vi "Filters_on_Single_Frame_Displacements-2.vi"(5 "[IN] Possibly\nMoving (X,Y)":dbl[][](array[numeric]), 6 "Areas of\nobjects":dbl[][](array[numeric]), 7 "[IN] Primary \nCoordinates (X,Y)":dbl[][](array[numeric]), 8 "error IN":errorcluster, 9 "% DIfference between \nParticle Squares":dbl, 10 "[IN] Dot matrix with \nstatuses for  potentially \nmoving dots":i16[][](array[numeric]), 11 "[IN] Potential\ndisplacement \n(X,Y,dX,dY)":dbl[][](array[numeric])) -> (0 "error OUT":errorcluster, 2 "[OUT] Dot matrix with \nstatuses for potentially \nmoving dots":i16[][](array[numeric]), 3 "[OUT] Filtered\ndisplacements":dbl[][](array[numeric]))   [LabVIEW 2013]
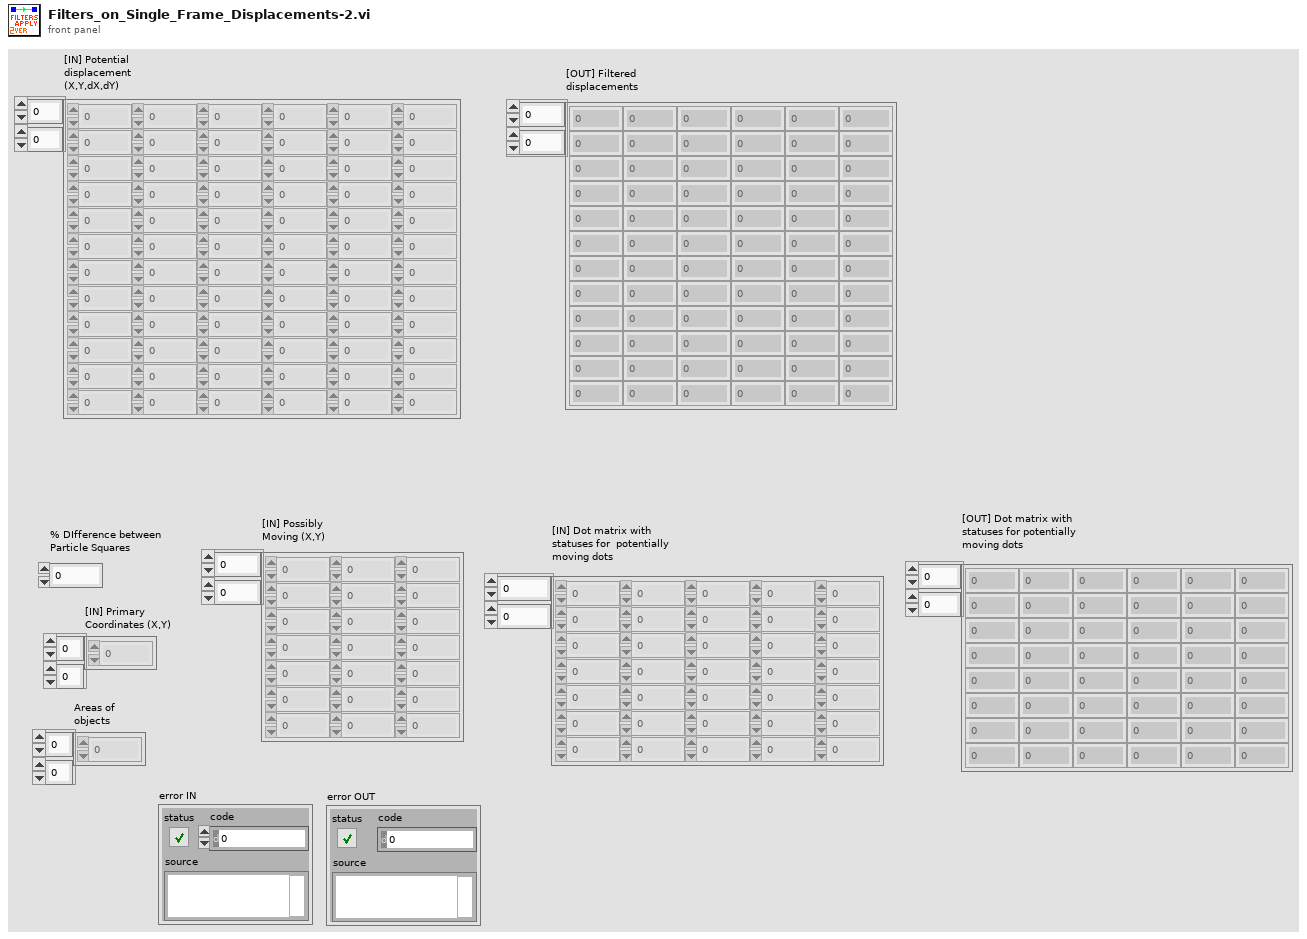
[diagram p1: front panel]
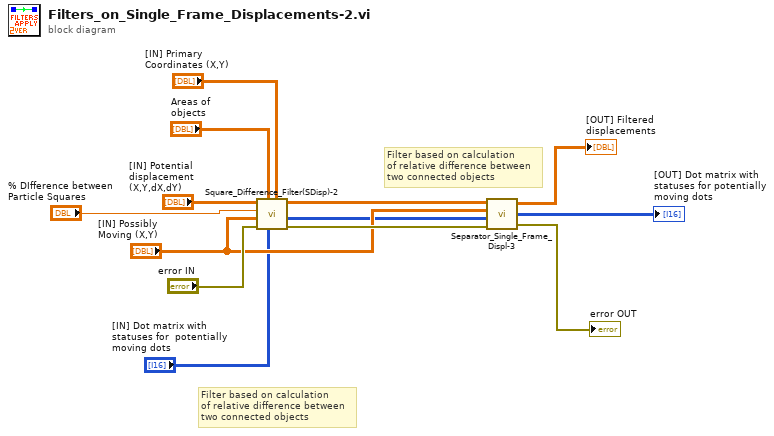
[diagram p0: block diagram]
diagram:
  # "Filter based on calculation \nof relative difference between\ntwo connected objects"
  # "Filter based on calculation \nof relative difference between\ntwo connected objects"
  n1 = call "Square_Difference_Filter(SDisp)-2.vi"("X,Y"="[IN] Primary \nCoordinates (X,Y)", "[IN] Dot matrix with \nstatuses for potentially \nmoving dots"="[IN] Dot matrix with \nstatuses for  potentially \nmoving dots", "Areas"="Areas of\nobjects", "error IN"="error IN", "[IN] Possibly\nMoving (X,Y)"="[IN] Possibly\nMoving (X,Y)", "% DIfference between \nParticle Squares"="% DIfference between \nParticle Squares", "(X,Y,dX,dY) In"="[IN] Potential\ndisplacement \n(X,Y,dX,dY)") -> ("error OUT"=w7:errorcluster, "[OUT] Dot matrix with \nstatuses after searching \nof unmoving dots"=w2:i16[][], "[OUT] Filtered Single Displ (X,Y,dX,dY)"=w8:dbl[][])  [unwired: 2 in]
  n2 = call "Separator_Single_Frame_Displ-3.vi"("error IN"=w7, "[IN] Dot matrix with \nstatuses for potentially \nmoving dots"=w2, "[IN] Possibly\nMoving (X,Y)"="[IN] Possibly\nMoving (X,Y)", "[IN] Single Displ"=w8) -> ("error OUT"=→"error OUT":errorcluster, "[OUT] Dot matrix with \nstatuses for potentially \nmoving dots"=→"[OUT] Dot matrix with \nstatuses for potentially \nmoving dots":i16[][], "[OUT] Single Displ\nw/t problems"=→"[OUT] Filtered\ndisplacements":dbl[][])
